vi "Write Is Interface.vi"(8 "error in (no error)":errorcluster, 10 "Is Interface":bool, 11 "Class in":refnum<class "Class.lvclass">) -> (0 "error out":errorcluster, 3 "Class out":refnum<class "Class.lvclass">)   [LabVIEW 2021, in "TAF Proj Document Type.lvlib" / "Class.lvclass"]
uses:
  <vilib>/Wovalab/AntiDoc/Document Type/Add-ons/LabVIEW TAF Project/Class/Class.lvclass
  <vilib>/Wovalab/AntiDoc/Document Type/Add-ons/LabVIEW TAF Project/Class/Class.lvclass/Class.ctl
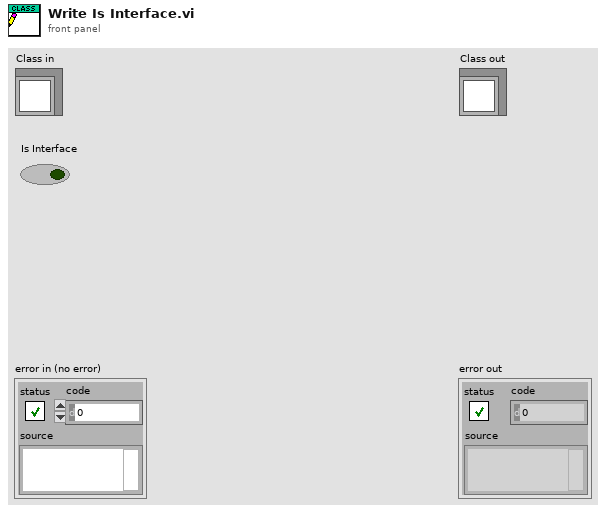
[diagram p1: front panel]
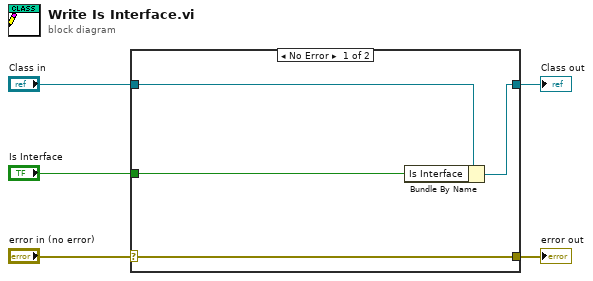
[diagram p0: block diagram]
diagram:
  n1 = case shown="No Error" "error in (no error)" {
    selector: "error in (no error)" -> [w9 w10]
    tunnel: [w9 w10] -> w4
    tunnel: [w7 w11] -> w2
    tunnel: "Class in" -> [w8 w11]
    tunnel: "Is Interface" -> [w6 _]
    frame No Error {
      n2 = Bundle By Name(cluster=w8, "Is Interface"=w6) -> (w7:refnum<class "Class.lvclass">)
    }
    frame Error {
    }
  }
  "error out" <- w4
  "Class out" <- w2
